vi "state machie.vi"   [LabVIEW 2022 SP3]
types:
  T1 = enum16{"Intialize", "Process", "Macro Exit", "Exit"}
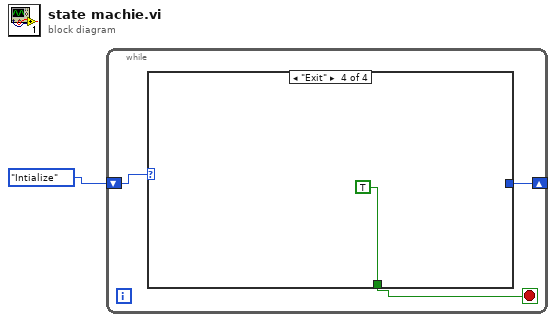
[diagram p0: block diagram]
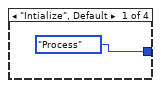
[diagram p2: hidden frame]
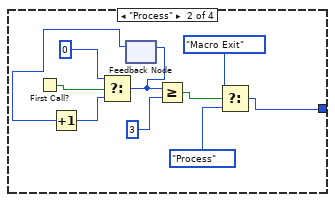
[diagram p3: hidden frame]
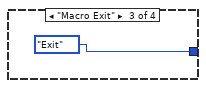
[diagram p4: hidden frame]
diagram:
  n1 = while {
    shift-right: [w3] -> _
    shift-left: T1."Intialize" -> [w4]
    stop <- w2 stop-if-true
    n2 = case shown="\"Exit\"" w4 {
      tunnel: [T1."Process" w6 T1."Exit" _] -> w3
      tunnel: [_ _ _ TRUE] -> w2
      frame "Intialize", Default {
      }
      frame "Process" {
        n3 = First Call?() -> (First Call?: T/F=w15:bool)
        n4 = feedback #1() -> (w11:i32)  [unwired: 1 in]
        n5 = Increment(x=w11) -> (x+1=w10:i32)
        n6 = Select(t=0, s=w15, f=w10) -> (s? t:f=w12:i32)
        n7 = feedback-in #1(w12) -> ()
        n8 = Greater Or Equal?(x=w12, y=3) -> (x >= y?=w9:bool)
        n9 = Select(t=T1."Macro Exit", s=w9, f=T1."Process") -> (s? t:f=w6:T1)
      }
      frame "Macro Exit" {
      }
      frame "Exit" {
      }
    }
  }
